vi "Upload from String.vi"(8 "error in":errorcluster, 9 "Multiplexer":cluster{"Index":string, "Sub-Index":string}, 10 "Node-ID":u8, 11 "CANopen Master in":refnum<class "CANopen Master.lvclass">) -> (0 "error out":errorcluster, 1 "Value":u8[](array[numeric]), 2 "Success?":bool, 3 "CANopen Master out":refnum<class "CANopen Master.lvclass">)   [LabVIEW 2024, in "CANopen Master.lvlib" / "CANopen Master.lvclass"]
uses:
  CANopen Master.lvclass
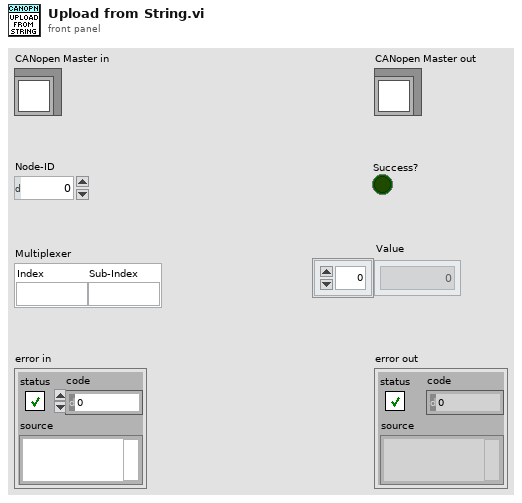
[diagram p1: front panel]
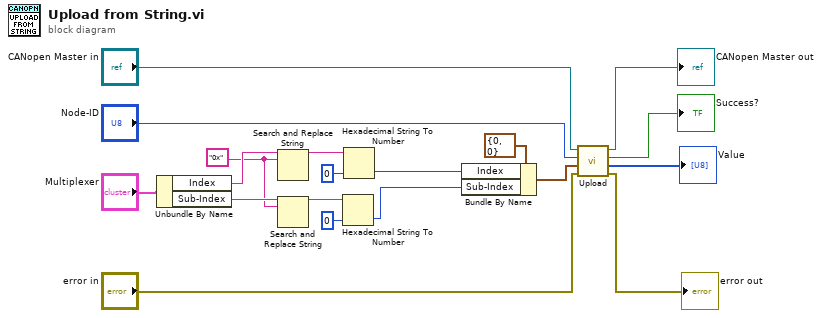
[diagram p0: block diagram]
diagram:
  w1 = "0x" ("search string")
  n1 = Unbundle By Name("Multiplexer") -> ("Index"=w7:string, "Sub-Index"=w6:string)
  n2 = Search and Replace String(input string=w7, search string=w1) -> (result string=w3:string)  [unwired: 6 in, 3 out]
  n3 = Search and Replace String(input string=w6, search string=w1) -> (result string=w2:string)  [unwired: 6 in, 3 out]
  n4 = Hexadecimal String To Number(string=w2, default (0uL)=u8 0 ("default (0 U32)")) -> (number=w9:u8)  [unwired: 1 in, 1 out]
  n5 = Hexadecimal String To Number(string=w3, default (0uL)=u16 0 ("default (0 U32)")) -> (number=w10:u16)  [unwired: 1 in, 1 out]
  n6 = Bundle By Name(cluster=cluster{"Index":u16, "Sub-Index":u8} {"Index"=0, "Sub-Index"=0} ("Multiplexer"), "Index"=w10, "Sub-Index"=w9) -> (w12:cluster{"Index":u16, "Sub-Index":u8})
  n7 = call "Upload.vi"("error in"="error in", "Multiplexer"=w12, "Node-ID"="Node-ID", "CANopen Master in"="CANopen Master in") -> ("error out"=→"error out":errorcluster, "Value"=→"Value":u8[], "Success?"=→"Success?":bool, "CANopen Master out"=→"CANopen Master out":refnum<class "CANopen Master.lvclass">)  [unwired: 4 in]
